vi "Get 007 Money.vi"(8 "Error In":errorcluster, 10 "007 Data":T1, 11 "Player Money":string[](array[string])) -> (0 "Error Out":errorcluster, 3 "007 Data Out":T1)   [LabVIEW 2015]
uses:
  007 Data.ctl
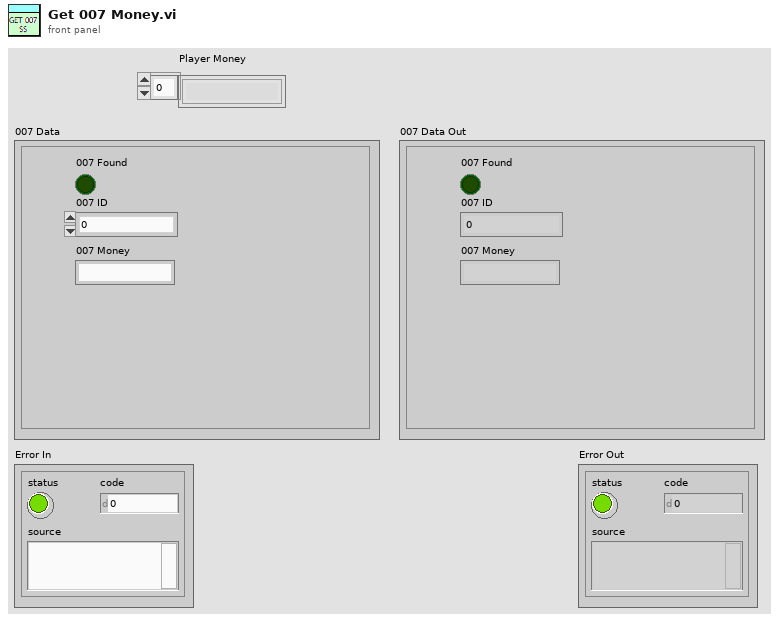
[diagram p1: front panel]
types:
  T1 = typedef "007 Data.ctl" = cluster{"007 ID":dbl, "007 Found":bool, "007 Money":string}
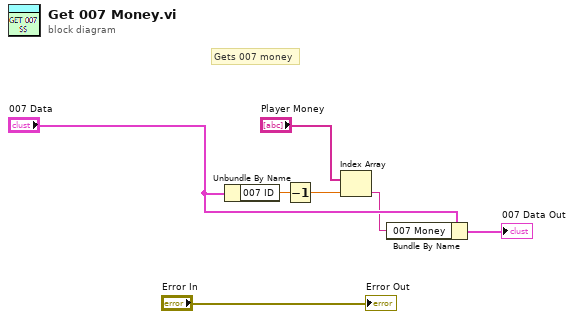
[diagram p0: block diagram]
diagram:
  # "Gets 007 money"
  n1 = Unbundle By Name("007 Data") -> ("007 ID"=w3:dbl)
  n2 = Decrement(x=w3) -> (x-1=w7:dbl)
  n3 = Index Array(array="Player Money", index=w7) -> (element=w4:string)
  n4 = Bundle By Name(cluster="007 Data", "007 Money"=w4) -> (→"007 Data Out":T1)
  "Error Out" <- "Error In"
